vi "Reset Benchmarks.vi"(8 "error in (no error)":errorcluster, 11 "CIFChannels in":refnum<class "CIFChannels.lvclass">) -> (0 "error out":errorcluster, 3 "CIFChannels out":refnum<class "CIFChannels.lvclass">)   [LabVIEW 2021, in "CIFChannels.lvclass"]
uses:
  CIFChannels.lvclass
  CIFChannels.lvclass/CIFChannels.ctl
  <vilib>/CIF Foundation/CIF Utilities/Statistics/I64/Stats_I64_CIF_U.lvclass/Stats_I64_CIF_U.ctl
  <vilib>/CIF Foundation/CIF Utilities/Statistics/I64/Data Accessors/Read Max History.vi
  <vilib>/CIF Foundation/CIF Utilities/Statistics/I64/Stats_I64_CIF_U.lvclass
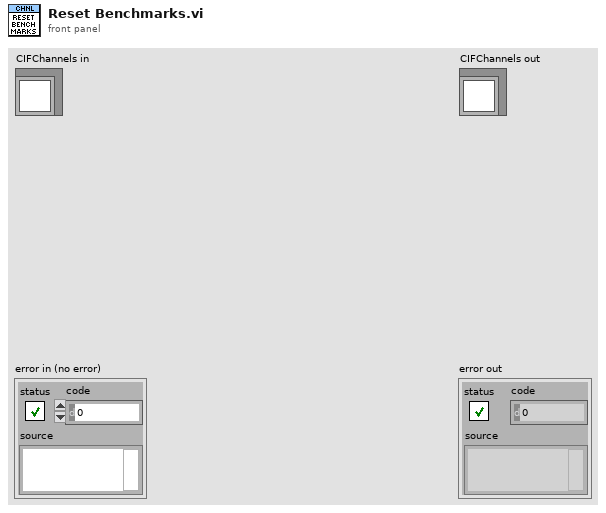
[diagram p1: front panel]
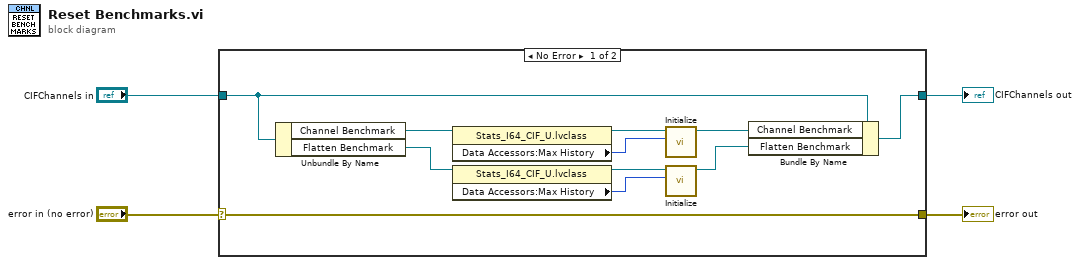
[diagram p0: block diagram]
diagram:
  n1 = case shown="No Error" "error in (no error)" {
    selector: "error in (no error)" -> [w15 w17]
    tunnel: [w15 w17] -> w3
    tunnel: [w13 w16] -> w1
    tunnel: "CIFChannels in" -> [w14 w16]
    frame No Error {
      n2 = Unbundle By Name(w14) -> ("Channel Benchmark"=w7:refnum<class "Stats_I64_CIF_U.lvclass">, "Flatten Benchmark"=w12:refnum<class "Stats_I64_CIF_U.lvclass">)
      n3 = property class="Stats_I64_CIF_U.lvclass"(reference=w7) -> (reference out=w6:refnum<class "Stats_I64_CIF_U.lvclass">, "Data Accessors:Max History"=w8:i32)  [unwired: 1 in, 1 out]
      n4 = property class="Stats_I64_CIF_U.lvclass"(reference=w12) -> (reference out=w11:refnum<class "Stats_I64_CIF_U.lvclass">, "Data Accessors:Max History"=w10:i32)  [unwired: 1 in, 1 out]
      n5 = call <vilib>:"Initialize.vi"("Max History"=w8, "Stats_I64_CIF_U in"=w6) -> ("Stats_I64_CIF_U out"=w5:refnum<class "Stats_I64_CIF_U.lvclass">)  [unwired: 8 in, 1 out]
      n6 = call <vilib>:"Initialize.vi"("Max History"=w10, "Stats_I64_CIF_U in"=w11) -> ("Stats_I64_CIF_U out"=w9:refnum<class "Stats_I64_CIF_U.lvclass">)  [unwired: 8 in, 1 out]
      n7 = Bundle By Name(cluster=w14, "Channel Benchmark"=w5, "Flatten Benchmark"=w9) -> (w13:refnum<class "CIFChannels.lvclass">)
    }
    frame Error {
    }
  }
  "error out" <- w3
  "CIFChannels out" <- w1
